vi "PXI-2510 Main Page.vi"(8 "error in (no error)":errorcluster, 11 "Node Ptr":T1 format="%.0x") -> (0 "error out":errorcluster)   [LabVIEW 2011, in "PXI-2510 Custom Device.lvlib"]
uses:
  PXI-2510 Custom Device.lvlib
  <vilib>/NI Veristand/Custom Device API/Custom Device Item Ref.ctl
  FIU Global Strings.vi
  <vilib>/NI Veristand/Custom Device API/Get Item Property (String).vi
  <vilib>/NI Veristand/Custom Device API/Set Item Property (String).vi
  <vilib>/NI Veristand/Custom Device API/Custom Device API.lvlib
panel:
  in  "Hardware Device Name":string caption="This is the device name which appears \nin Measurement and Automation\n Explorer (MAX)"
  in  "Header":cluster{"Section Name":string}={"Section Name"="Custom Device Item Settings"}
  in  "Description":string
  in  "Name":string
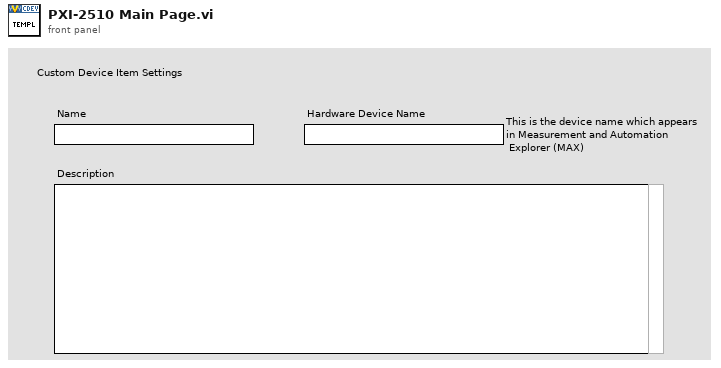
[diagram p1: front panel]
types:
  T1 = typedef "Custom Device API.lvlib/Custom Device Item Ref.ctl" = u64
  T2 = typedef "Custom Device API.lvlib/Custom Device Item Info.ctl" = cluster{"Name":string, "Is Channel":bool, "GUID":string}
  T3 = typedef "Custom Device API.lvlib/Custom Device Commands.ctl" = enum16{"Default", "Item renamed", "Shutdown", "Dynamic button pressed"}
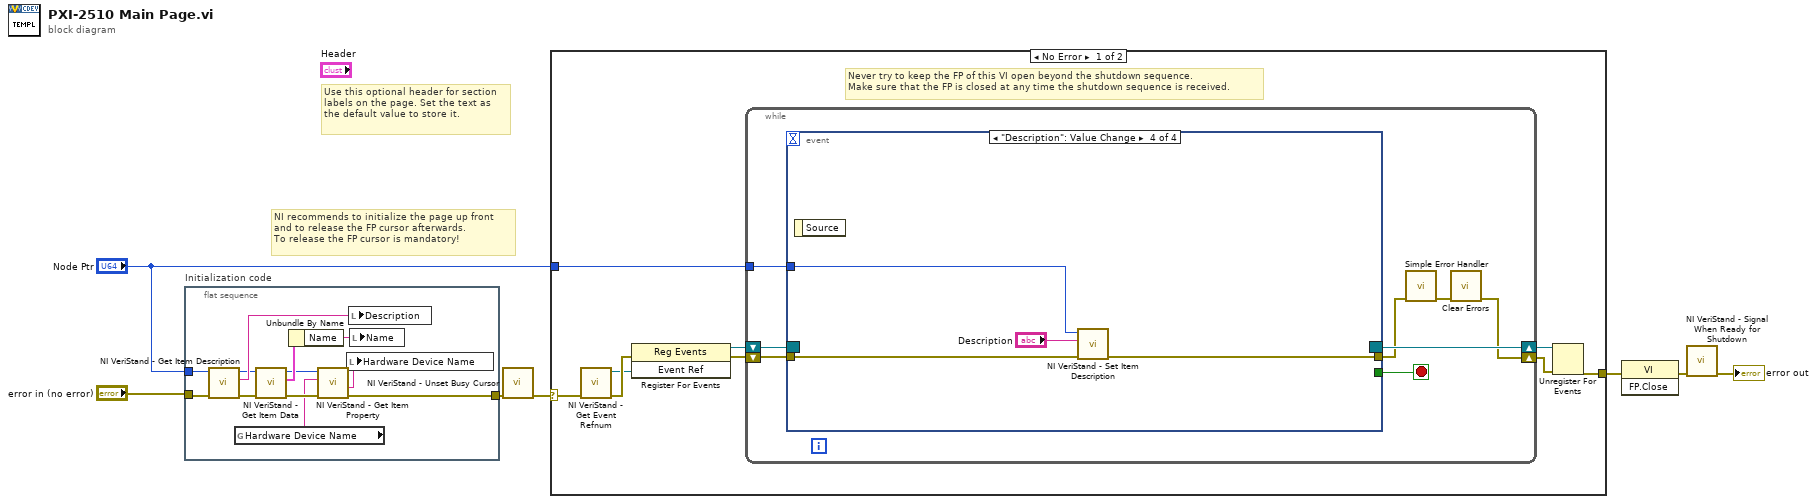
[diagram p0: block diagram]
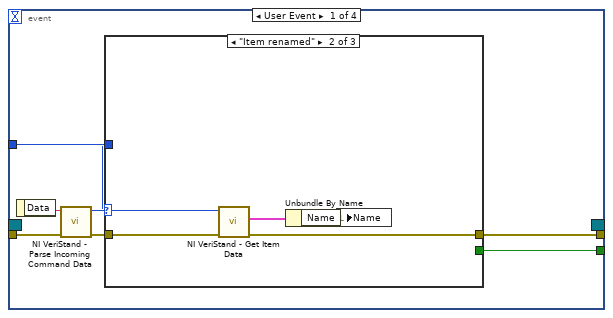
[diagram p2: hidden frame]
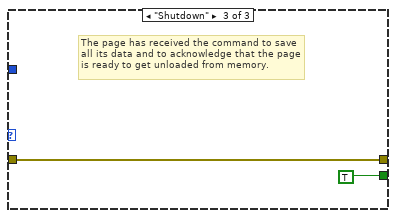
[diagram p4: hidden frame]
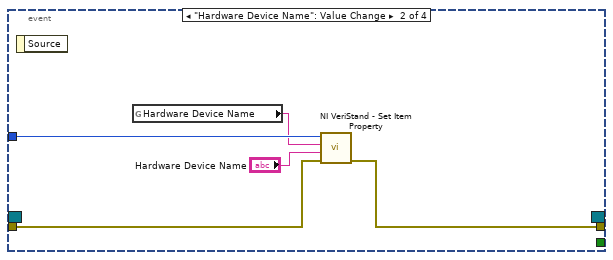
[diagram p5: hidden frame]
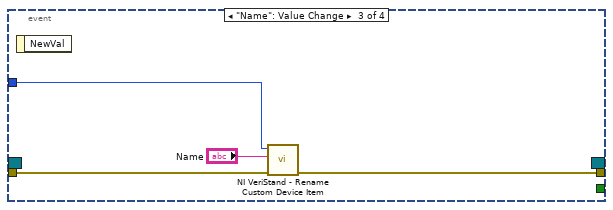
[diagram p6: hidden frame]
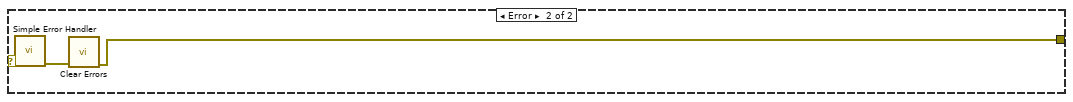
[diagram p7: hidden frame]
diagram:
  # "Use this optional header for section labels on the page. Set the text as the default value to store it."
  # "NI recommends to initialize the page up front\nand to release the FP cursor afterwards.\nTo release the FP cursor is mandatory!"
  n1 = flat-sequence "Initialization code" {
    tunnel: "error in (no error)" -> [w19]
    tunnel: "Node Ptr" -> [w18]
    tunnel: [w10] -> w2
    frame #0 {
      n2 = call <vilib>:"NI VeriStand - Get Item Description.vi"("error in (no error)"=w19, "Item Ref in"=w18) -> ("error out"=w16:errorcluster, "Description"=w17:string, "Item Ref out"=w15:T1)  [unwired: 7 out]
      n3 = global read "FIU Global Strings.vi" "Hardware Device Name"() -> (w8:string)
      n4 = call <vilib>:"NI VeriStand - Get Item Data.vi"("error in (no error)"=w16, "Item Ref in"=w15) -> ("error out"=w9:errorcluster, "Item Info"=w14:T2, "Item Ref out"=w12:T1)  [unwired: 7 out]
      n5 = Unbundle By Name(w14) -> ("Name"=w13:string)
      n6 = call-poly <vilib>:"NI VeriStand - Get Item Property.vi"("error in (no error)"=w9, "Property Name"=w8, "Item Ref in"=w12) -> ("error out"=w10:errorcluster, "Value"=w11:string)  [unwired: 5 in, 2 out]
      n7 = local write "Hardware Device Name"(w11) -> ()
      n8 = local write "Description"(w17) -> ()
      n9 = local write "Name"(w13) -> ()
    }
  }
  n10 = call <vilib>:"NI VeriStand - Unset Busy Cursor.vi"("error in (no error)"=w2) -> ("error out"=w1:errorcluster)  [unwired: 10 out]
  n11 = case shown="No Error" w1 {
    selector: w1 -> [w20 w67]
    tunnel: [w25 w65] -> w5
    tunnel: "Node Ptr" -> [w21 _]
    frame No Error {
      # "Never try to keep the FP of this VI open beyond the shutdown sequence.\nMake sure that the FP is closed at any time the shutdown sequence is received."
      n12 = call <vilib>:"NI VeriStand - Get Event Refnum.vi"("error in (no error)"=w20) -> ("error out"=w28:errorcluster, "Event Ref"=w24:refnum<user-event>)  [unwired: 9 out]
      n13 = register-events(error in=w28, w24) -> (reference out=w22:refnum<event-registration>, error out=w23:errorcluster)  [unwired: 1 in]
      n14 = while {
        tunnel: w21 -> [w32]
        shift-right: [w29] -> w26
        shift-left: w23 -> [w35]
        shift-right: [w36] -> w27
        shift-left: w22 -> [w34]
        stop <- w33 stop-if-true
        n15 = event shown="[3] \"Description\": Value Change" {
          selector: w34 -> [_ _ _ _]
          dyn-events: [_ _ _ _] -> w36
          timeout: _ -> [_ _ _ _]
          tunnel: w35 -> [w43 w54 w60 w63]
          tunnel: [w39 _ _ _] -> w33
          tunnel: [w38 w53 w59 w62] -> w31
          tunnel: w32 -> [w37 w56 w58 w64]
          event User Event {
            n16 = event-data() -> ("Data"=w42:string)  [unwired: 1 out]
            n17 = call <vilib>:"NI VeriStand - Parse Incoming Command Data.vi"("error in (no error)"=w43, "Incoming data"=w42) -> ("error out"=w41:errorcluster, "Action"=w40:T3)  [unwired: 8 out]
            n18 = case shown="\"Item renamed\"" w40 {
              tunnel: w41 -> [w44 w49 w50]
              tunnel: [_ _ TRUE] -> w39
              tunnel: [w44 w46 w50] -> w38
              tunnel: w37 -> [_ w48 _]
              frame "Default", Default {
              }
              frame "Item renamed" {
                n19 = call <vilib>:"NI VeriStand - Get Item Data.vi"("error in (no error)"=w49, "Item Ref in"=w48) -> ("error out"=w46:errorcluster, "Item Info"=w47:T2)  [unwired: 8 out]
                n20 = Unbundle By Name(w47) -> ("Name"=w45:string)
                n21 = local write "Name"(w45) -> ()
              }
              frame "Shutdown" {
                # "The page has received the command to save all its data and to acknowledge that the page is ready to get unloaded from memory."
              }
            }
          }
          event "Hardware Device Name": Value Change {
            n22 = event-data() -> ()  [unwired: 2 out]
            n23 = global read "FIU Global Strings.vi" "Hardware Device Name"() -> (w52:string)
            n24 = call-poly <vilib>:"NI VeriStand - Set Item Property.vi"("error in (no error)"=w54, "Value"="Hardware Device Name", "Property Name"=w52, "Item Ref in"=w56) -> ("error out"=w53:errorcluster)  [unwired: 5 in, 2 out]
          }
          event "Name": Value Change {
            n25 = event-data() -> ()  [unwired: 2 out]
            n26 = call <vilib>:"NI VeriStand - Rename Custom Device Item.vi"("error in (no error)"=w60, "New Name"="Name", "Item Ref in"=w58) -> ("error out"=w59:errorcluster)  [unwired: 8 out]
          }
          event "Description": Value Change {
            n27 = event-data() -> ()  [unwired: 2 out]
            n28 = call <vilib>:"NI VeriStand - Set Item Description.vi"("error in (no error)"=w63, "Description"="Description", "Item Ref in"=w64) -> ("error out"=w62:errorcluster)  [unwired: 8 out]
          }
        }
        n29 = call <vilib>:"Simple Error Handler.vi"("error in (no error)"=w31) -> ("error out"=w30:errorcluster)  [unwired: 1 in, 7 out]
        n30 = call <vilib>:"Clear Errors.vi"("error in (no error)"=w30) -> ("error out"=w29:errorcluster)  [unwired: 6 out]
      }
      n31 = Unregister For Events(event registration refnum=w27, error in=w26) -> (error out=w25:errorcluster)
    }
    frame Error {
      n32 = call <vilib>:"Simple Error Handler.vi"("error in (no error)"=w67) -> ("error out"=w66:errorcluster)  [unwired: 1 in, 7 out]
      n33 = call <vilib>:"Clear Errors.vi"("error in (no error)"=w66) -> ("error out"=w65:errorcluster)  [unwired: 6 out]
    }
  }
  n34 = invoke class="VI" method="FP.Close"(error in=w5) -> (error out=w4:errorcluster)  [unwired: 2 in, 2 out]
  n35 = call <vilib>:"NI VeriStand - Signal When Ready for Shutdown.vi"("error in (no error)"=w4) -> ("error out"=→"error out":errorcluster)  [unwired: 10 out]
